vi "Monitor_clear.vi"(8 "error in":errorcluster, 11 "Tab Control":refnum<vi>) -> (0 "error out":errorcluster)   [LabVIEW 2015]
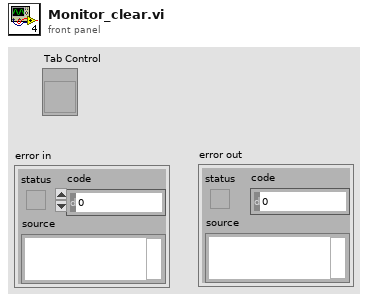
[diagram p1: front panel]
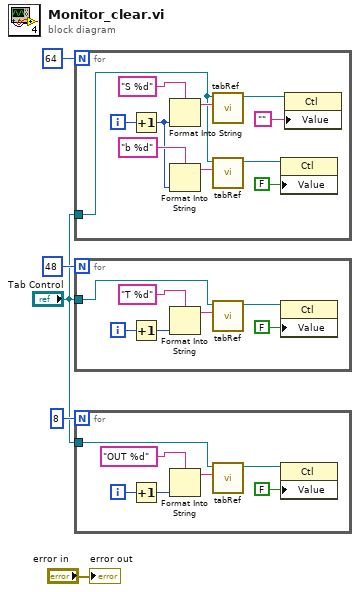
[diagram p0: block diagram]
diagram:
  n1 = for {
    N: 64 -> [_]
    tunnel: "Tab Control" -> [w6]
    i -> [w12]
    n2 = Increment(x=w12) -> (x+1=w9:i32)
    n3 = Format Into String(format string="S %d", w9) -> (resulting string=w8:string)  [unwired: 2 in, 1 out]
    n4 = Format Into String(format string="b %d", w9) -> (resulting string=w11:string)  [unwired: 2 in, 1 out]
    n5 = call "tabRef.vi"("control name"=w8, "Tab Control"=w6) -> ("control refnum"=w16:refnum<vi>)  [unwired: 8 in, 1 out]
    n6 = call "tabRef.vi"("control name"=w11, "Tab Control"=w6) -> ("control refnum"=w14:refnum<vi>)  [unwired: 8 in, 1 out]
    n7 = property class="Ctl"(reference=w14, "Value"=FALSE) -> ()  [unwired: 1 in, 2 out]
    n8 = property class="Ctl"(reference=w16, "Value"="") -> ()  [unwired: 1 in, 2 out]
  }
  n9 = for {
    N: 48 -> [_]
    tunnel: "Tab Control" -> [w20]
    i -> [w18]
    n10 = Increment(x=w18) -> (x+1=w17:i32)
    n11 = Format Into String(format string="T %d", w17) -> (resulting string=w23:string)  [unwired: 2 in, 1 out]
    n12 = call "tabRef.vi"("control name"=w23, "Tab Control"=w20) -> ("control refnum"=w22:refnum<vi>)  [unwired: 8 in, 1 out]
    n13 = property class="Ctl"(reference=w22, "Value"=FALSE) -> ()  [unwired: 1 in, 2 out]
  }
  n14 = for {
    N: 8 -> [_]
    tunnel: "Tab Control" -> [w27]
    i -> [w25]
    n15 = Increment(x=w25) -> (x+1=w24:i32)
    n16 = Format Into String(format string="OUT %d", w24) -> (resulting string=w30:string)  [unwired: 2 in, 1 out]
    n17 = call "tabRef.vi"("control name"=w30, "Tab Control"=w27) -> ("control refnum"=w29:refnum<vi>)  [unwired: 8 in, 1 out]
    n18 = property class="Ctl"(reference=w29, "Value"=FALSE) -> ()  [unwired: 1 in, 2 out]
  }
  "error out" <- "error in"
